vi "YKMW100 Computation Control.vi"(0 "VISA session":refnum<visa-resource-name>="MW100", 2 "Semiphore":T1, 5 "Mode":T2(ring), 11 "error in (no error)":errorcluster) -> (4 "dup VISA session":refnum<visa-resource-name>="MW100", 15 "error out":errorcluster)   [LabVIEW 2009]
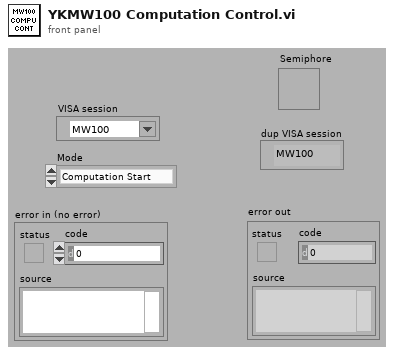
[diagram p1: front panel]
types:
  T1 = typedef "Semaphore RefNum" = refnum<k1>
  T2 = enum16{"Computation Start", "Computation stop", "Reset Computation", "Clear Computation"}
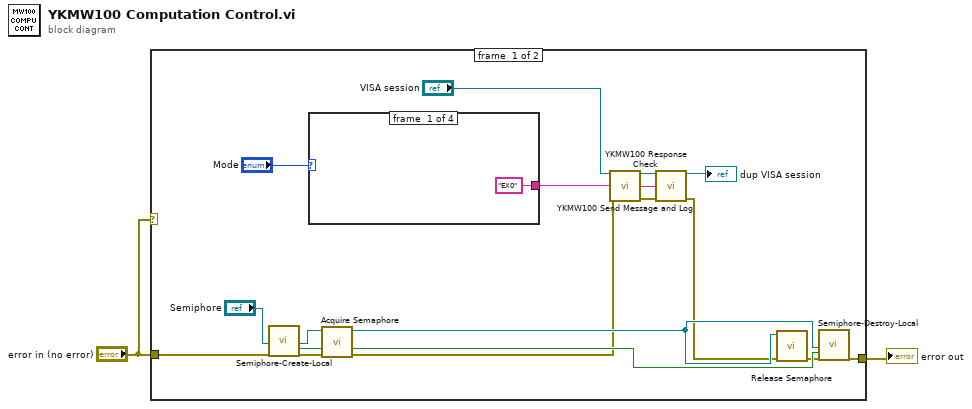
[diagram p0: block diagram]
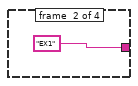
[diagram p2: hidden frame]
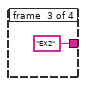
[diagram p3: hidden frame]
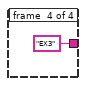
[diagram p4: hidden frame]
diagram:
  n1 = case shown="Error" "error in (no error)" {
    tunnel: "error in (no error)" -> [w6 w24]
    tunnel: [w3 w24] -> w2
    frame #0 {
      n2 = call "Semiphore-Create-Local.vi"("Semiphore"="Semiphore", "error in (no error)"=w6) -> ("semaphore"=w11:T1, "Local?"=w8:bool, "error out"=w10:errorcluster)  [unwired: 15 in]
      n3 = case shown="\"Computation Start\", Default" "Mode" {
        tunnel: ["EX0" ("Send Message (\"\")") "EX1" ("Send Message (\"\")") "EX2" ("Send Message (\"\")") "EX3" ("Send Message (\"\")")] -> w14
        frame #0 {
        }
        frame #1 {
        }
        frame #2 {
        }
        frame #3 {
        }
      }
      n4 = call <vilib>:"Acquire Semaphore.vi"("error in (no error)"=w10, "semaphore"=w11) -> ("error out"=w5:errorcluster, "semaphore out"=w9:T1)  [unwired: 3 in, 1 out]
      n5 = call "YKMW100 Send Message and Log.vi"("VISA session"="VISA session", "Send Message (\"\")"=w14, "error in (no error)"=w5) -> ("dup VISA session"=w19:refnum<visa-resource-name>, "Read Buffer"=w17:string, "error out"=w18:errorcluster)  [unwired: 10 in]
      n6 = call "YKMW100 Response Check.vi"("VISA session"=w19, "Message In (\"\")"=w17, "error in (no error)"=w18) -> ("dup VISA session"=→"dup VISA session":refnum<visa-resource-name>, "error out"=w4:errorcluster)  [unwired: 8 in, 3 out]
      n7 = call <vilib>:"Release Semaphore.vi"("error in (no error)"=w4, "semaphore"=w9) -> ("error out"=w7:errorcluster)  [unwired: 4 in, 1 out]
      n8 = call "Semiphore-Destroy-Local.vi"("Semiphore"=w9, "Local?"=w8, "error in (no error)"=w7) -> ("error out"=w3:errorcluster)  [unwired: 16 in]
    }
    frame #1 {
    }
  }
  "error out" <- w2
